vi "Get UTC Offset.vi"(10 "time":timestamp) -> (1 "UTC Offset String":string, 2 "UTC Offset (seconds)":i32)   [LabVIEW 2011]
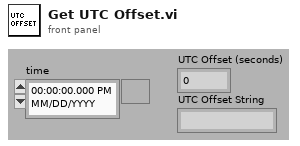
[diagram p1: front panel]
types:
  T1 = cluster{"second":i32, "minute":i32, "hour":i32, "day of month":i32, "month":i32, "year":i32, "day of week":i32, "day of year":i32, "is DST":i32}
  T2 = typedef "LVDateTimeRec.ctl" = cluster{"fractional second":dbl, "second":i32, "minute":i32, "hour":i32, "day of month":i32, "month":i32, "year":i32, "day of week":i32, "day of year":i32, "DST":i32}
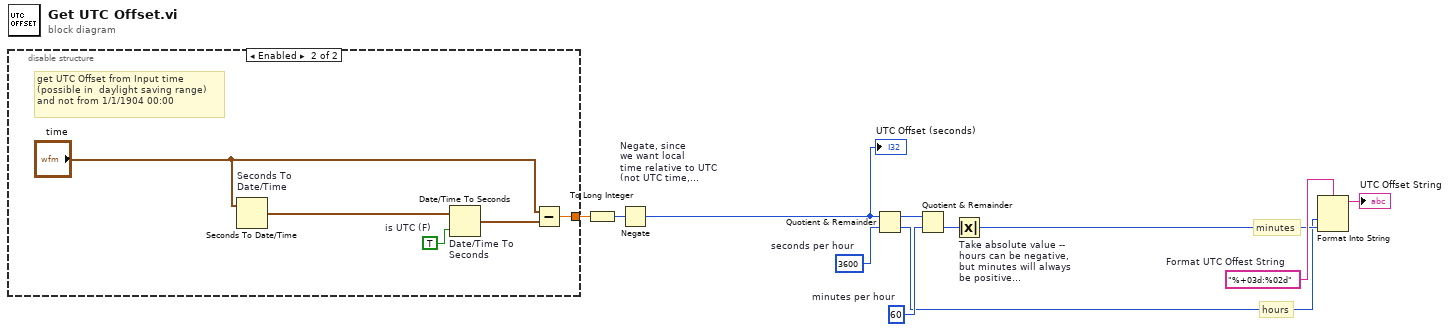
[diagram p0: block diagram]
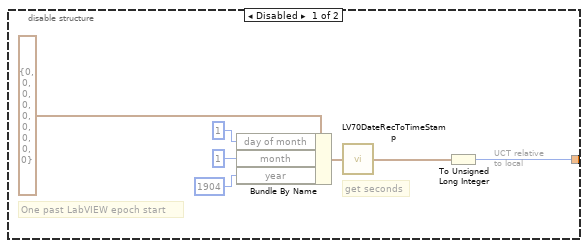
[diagram p2: hidden frame]
diagram:
  w7 = 60  # minutes per hour
  w9 = 3600  # seconds per hour
  w10 = "%+03d:%02d"  # Format UTC Offest String
  # "minutes"
  # "hours"
  n1 = disable-structure shown="Enabled" {
    disable-tunnel: [w18 w19] -> w11
    frame Disabled {
      # "One past LabVIEW epoch start"
      # "UCT relative to local"
      # "get seconds"
      n2 = Bundle By Name(cluster=T1 {"second"=0, "minute"=0, "hour"=0, "day of month"=0, "month"=0, "year"=0, "day of week"=0, "day of year"=0, "is DST"=0} ("date time rec"), "day of month"=1, "month"=1, "year"=1904) -> (w12:T1)
      n3 = call <vilib>:"LV70DateRecToTimeStamp.vi"("date time rec"=w12) -> ("Time Stamp"=w17:timestamp)
      n4 = To Unsigned Long Integer(number=w17) -> (unsigned 32bit integer=w18:u32)
    }
    frame Enabled {
      w22 = TRUE  # is UTC (F)
      # "get UTC Offset from Input time\n(possible in  daylight saving range) \nand not from 1/1/1904 00:00"
      n5 = Seconds To Date/Time "Seconds To \nDate/Time"(time stamp (now)="time") -> (date time rec=w23:T2)  [unwired: 1 in]
      n6 = Date/Time To Seconds "Date/Time To \nSeconds"(1:w22, 2:w23) -> (0:w20:timestamp)
      n7 = Subtract(x="time", y=w20) -> (x-y=w19:dbl)
    }
  }
  n8 = To Long Integer(number=w11) -> (32bit integer=w3:i32)
  n9 = Negate "Negate, since \nwe want local \ntime relative to UTC \n(not UTC time, \nrelative to local time)."(x=w3) -> (-x=w2:i32)
  "UTC Offset (seconds)" <- w2
  n10 = Quotient & Remainder(x=w2, y=w9) -> (x-y*floor(x/y)=w8:i32, floor(x/y)=w5:i32)
  n11 = Quotient & Remainder(x=w8, y=w7) -> (floor(x/y)=w4:i32)  [unwired: 1 out]
  n12 = Absolute Value "Take absolute value -- hours can be negative, \nbut minutes will always be positive \n(minutes is implicitly negative, if hours is negative)"(x=w4) -> (abs(x)=w6:i32)
  n13 = Format Into String(format string=w10, w5, w6) -> (resulting string=→"UTC Offset String":string)  [unwired: 2 in, 1 out]
